vi "SetFillLevel.vi"(0 "object in":refnum<class "CetoniPump.lvclass">, 2 "GoToLevelSettings":T1, 5 "error in (no error)":errorcluster) -> (14 "object out":refnum<class "CetoniPump.lvclass">, 16 "Values Not Permitted":bool, 17 "Coerced Level":dbl, 18 "Coerced Flow":dbl, 19 "error out":errorcluster)   [LabVIEW 2023, in "CetoniPump.lvclass"]
uses:
  CetoniPump.lvclass
  CetoniPump.lvclass/CetoniPump.ctl
  CETONI_SDK/lib/labview/labbCAN_Pump_API/labbCAN_Pump_API.lvlib
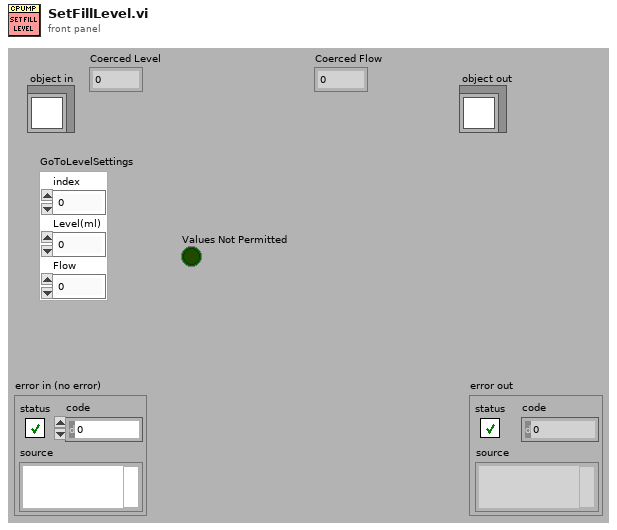
[diagram p1: front panel]
types:
  T1 = cluster{"index":i32, "Level(ml)":dbl, "Flow":dbl}
  T2 = cluster{"Pump Handle":i64, "Pump Name":string, "Maximum Volume":dbl, "Maximum Flow Rate":dbl, "Flow Rate":dbl, "Target Level":dbl, "Valve Handle":i64, "Has Valve?":bool, "Actual valve position":i32}[]
  T3 = cluster{"Pump Handle":i64, "Pump Name":string, "Maximum Volume":dbl, "Maximum Flow Rate":dbl, "Flow Rate":dbl, "Target Level":dbl, "Valve Handle":i64, "Has Valve?":bool, "Actual valve position":i32}
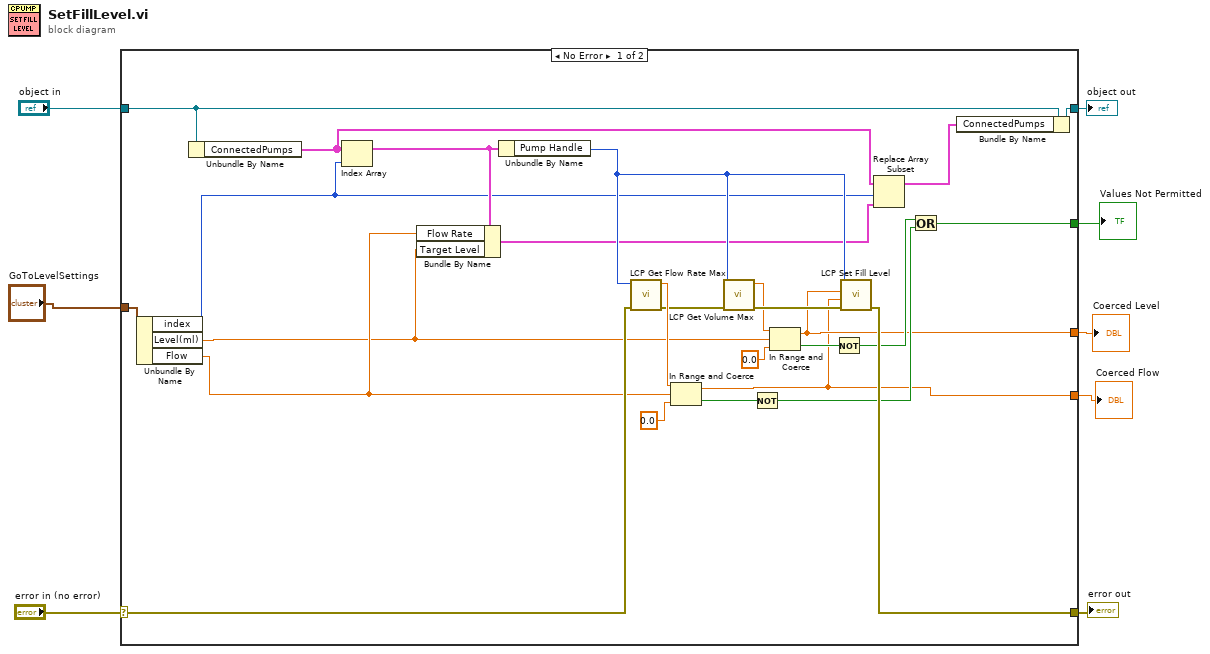
[diagram p0: block diagram]
diagram:
  n1 = case shown="No Error" "error in (no error)" {
    selector: "error in (no error)" -> [w30 w36]
    tunnel: [w33 w36] -> w7
    tunnel: [w16 w35] -> w5
    tunnel: "object in" -> [w34 w35]
    tunnel: [w20 _] -> w4
    tunnel: [w14 _] -> w3
    tunnel: [w13 _] -> w2
    tunnel: "GoToLevelSettings" -> [w12 _]
    frame No Error {
      n2 = Unbundle By Name(w12) -> ("index"=w11:i32, "Level(ml)"=w9:dbl, "Flow"=w10:dbl)
      n3 = Unbundle By Name(w34) -> ("ConnectedPumps"=w18:T2)
      n4 = Index Array(array=w18, index=w11) -> (element=w19:T3)
      n5 = Bundle By Name(cluster=w19, "Flow Rate"=w10, "Target Level"=w9) -> (w17:T3)
      n6 = Unbundle By Name(w19) -> ("Pump Handle"=w32:i64)
      n7 = call "LCP Get Flow Rate Max.vi"("error in (no error)"=w30, "Pump Handle"=w32) -> ("error out"=w29:errorcluster, "Maximum Flow Rate"=w31:dbl)  [unwired: 8 in]
      n8 = In Range and Coerce(upper limit=w31, x=w10, lower limit=0.0) -> (coerced(x)=w13:dbl, In Range?=w24:bool)
      n9 = call "LCP Get Volume Max.vi"("error in (no error)"=w29, "Pump Handle"=w32) -> ("error out"=w28:errorcluster, "Maximum Volume"=w27:dbl)  [unwired: 8 in]
      n10 = Not(x=w24) -> (.not. x?=w21:bool)
      n11 = In Range and Coerce(upper limit=w27, x=w9, lower limit=0.0) -> (coerced(x)=w14:dbl, In Range?=w23:bool)
      n12 = Not(x=w23) -> (.not. x?=w22:bool)
      n13 = call "LCP Set Fill Level.vi"("error in (no error)"=w28, "Flow"=w13, "Level"=w14, "Pump Handle"=w32) -> ("error out"=w33:errorcluster)  [unwired: 7 in]
      n14 = Replace Array Subset(array=w18, new element=w17, index=w11) -> (w15:T2)
      n15 = Or(x=w22, y=w21) -> (x .or. y?=w20:bool)
      n16 = Bundle By Name(cluster=w34, "ConnectedPumps"=w15) -> (w16:refnum<class "CetoniPump.lvclass">)
    }
    frame Error {
    }
  }
  "error out" <- w7
  "object out" <- w5
  "Values Not Permitted" <- w4
  "Coerced Level" <- w3
  "Coerced Flow" <- w2
